vi "지진 계측기 프로젝트.vi"() -> ()   [LabVIEW 2021]
uses:
  <vilib>/Utility/sysdir.llb/System Directory Type.ctl
  <vilib>/numeric/Random Number (Range) U64.vi
panel:
  out "지진센서값출력":u64(graph)
  in  "정지":bool
  in  "알람리셋":bool
  in  "감지시작":bool
  out "알림":bool
  out "출력메시지":string
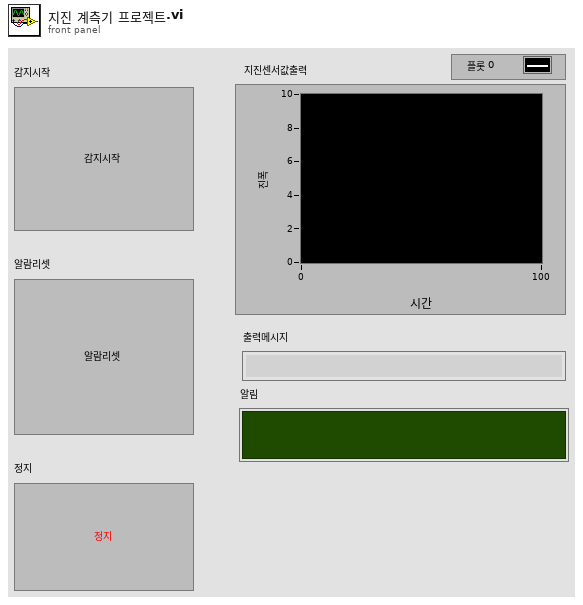
[diagram p1: front panel]
types:
  T1 = typedef "지진 계측기 상태 열거형 상수.ctl" = enum16{"초기화", "대기", "감지 시작", "알림 리셋", "정지"}
  T2 = cluster{"상태":T1, "알림":bool, "출력메시지":string, "지진센서값":dbl, "시간상수":i32}
  T3 = typedef "지진 계측기 상태 열거형 상수.ctl" = enum16{"초기화", "대기", "감지시작", "알람리셋", "정지", "파일저장"}
  T4 = enum16{"open", "replace", "create", "open or create", "replace or create", "replace or create with confirmation"}
  T5 = typedef "System Directory Type.ctl" = i32
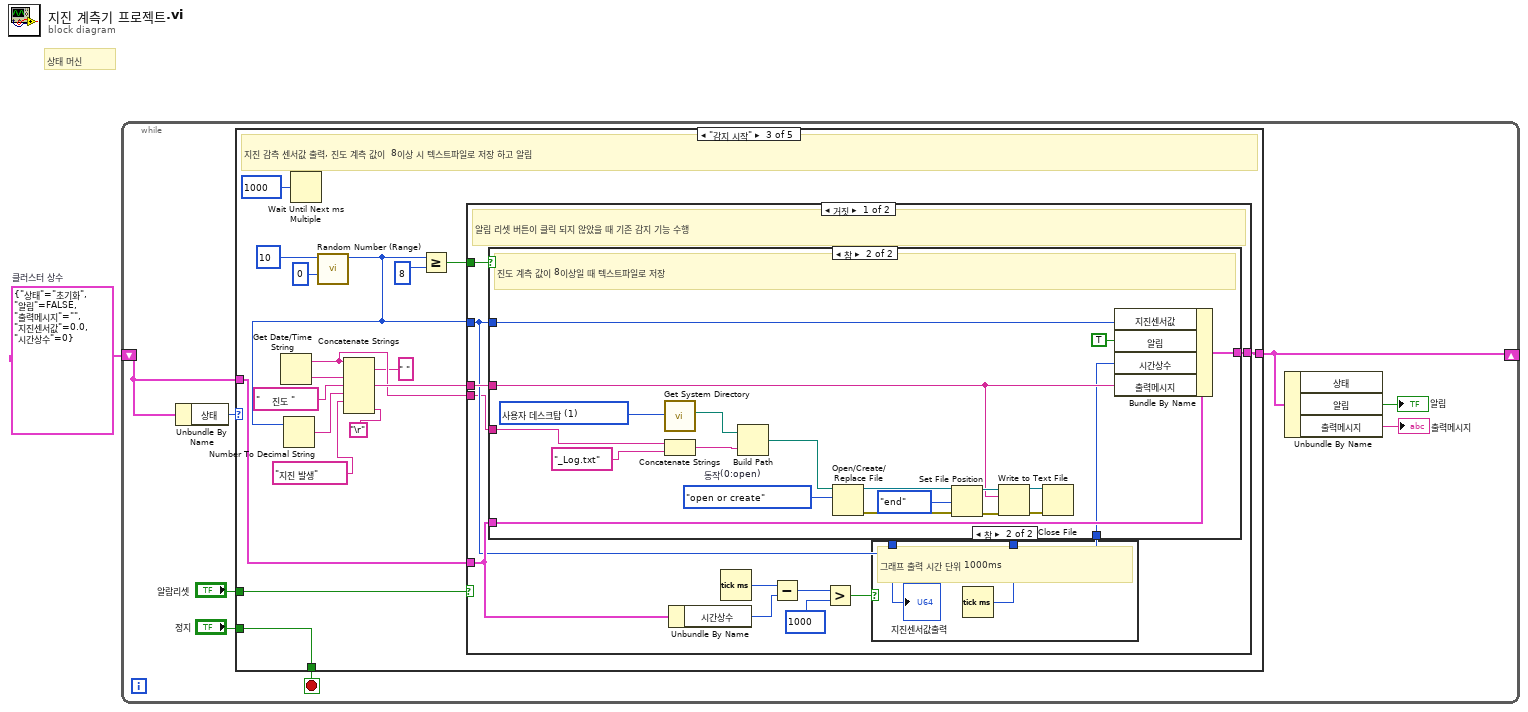
[diagram p0: block diagram]
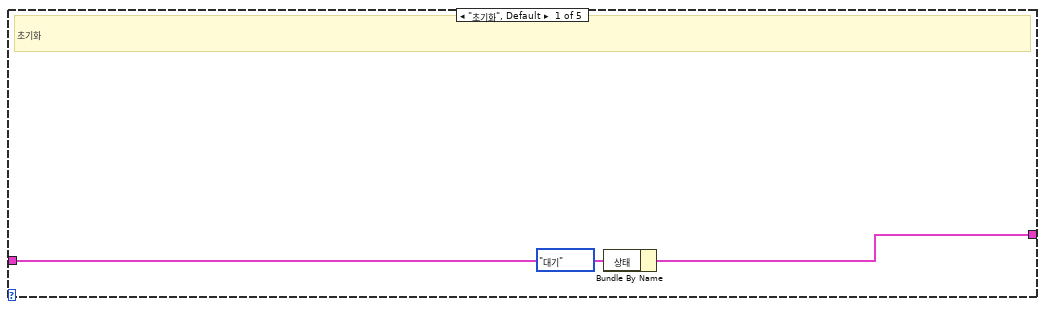
[diagram p2: hidden frame]
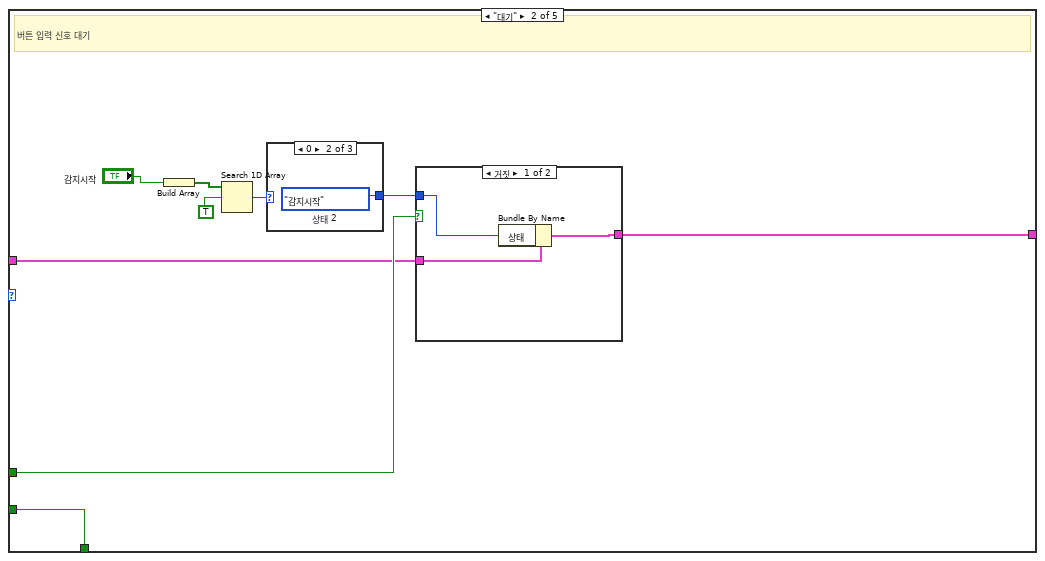
[diagram p3: hidden frame]
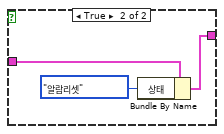
[diagram p4: hidden frame]
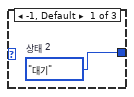
[diagram p5: hidden frame]
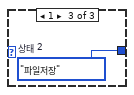
[diagram p6: hidden frame]
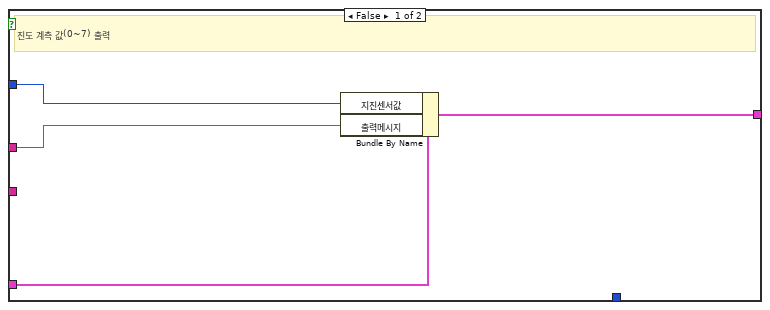
[diagram p8: hidden frame]
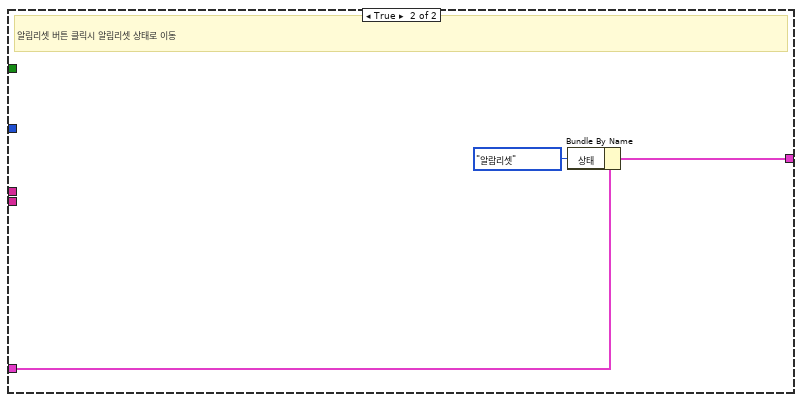
[diagram p9: hidden frame]
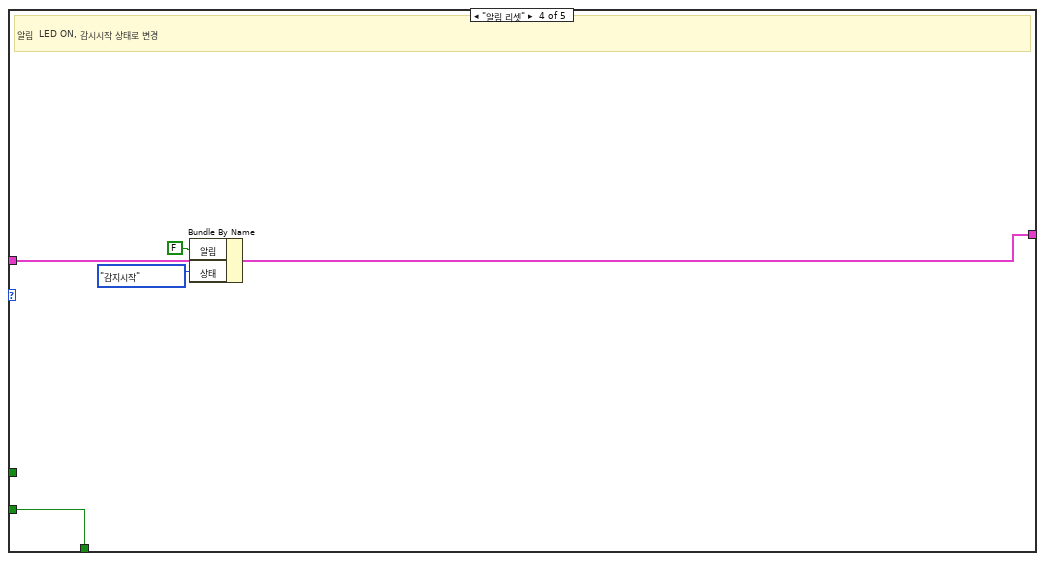
[diagram p10: hidden frame]
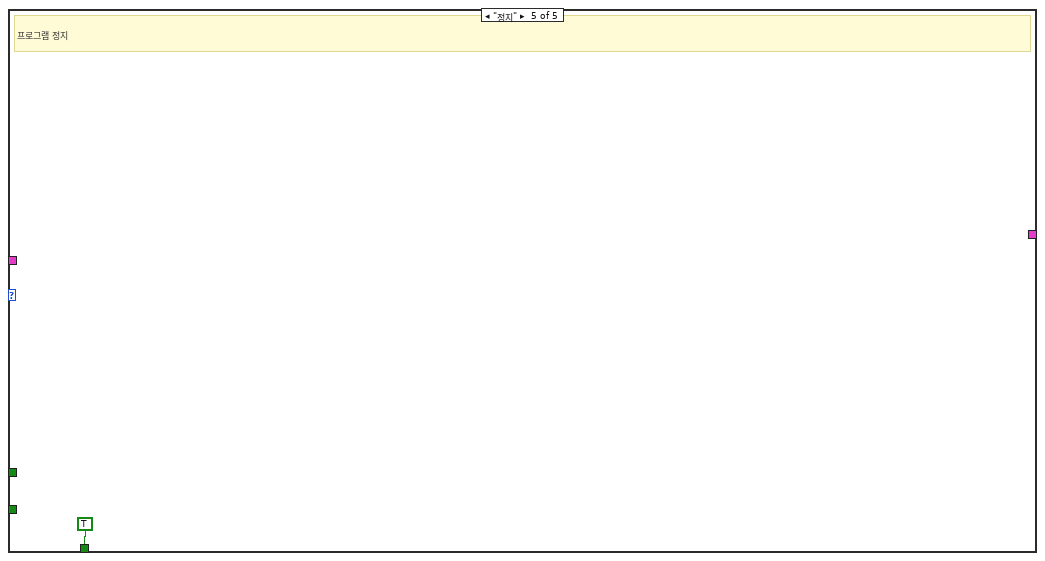
[diagram p11: hidden frame]
diagram:
  w1 = T2 {"상태"=enum."초기화", "알림"=FALSE, "출력메시지"="", "지진센서값"=0.0, "시간상수"=0}  # 클러스터 상수
  # "상태 머신"
  n1 = while {
    shift-right: [w8] -> _
    shift-left: w1 -> [w9]
    stop <- w7 stop-if-true
    n2 = Unbundle By Name(w9) -> ("상태"=w2:T1)
    n3 = case shown="\"감지 시작\"" w2 {
      tunnel: [w11 w15 w43 w91 _] -> w8
      tunnel: w9 -> [w12 w13 w42 w94 _]
      tunnel: [_ w14 w38 w90 TRUE] -> w7
      tunnel: "알람리셋" -> [_ w17 w41 _ _]
      tunnel: "정지" -> [_ w14 w38 w90 _]
      frame "초기화", Default {
        # "초기화"
        n4 = Bundle By Name(cluster=w12, "상태"=지진_계측기_상태_열거형_상수."대기") -> (w11:T2)
      }
      frame "대기" {
        # "버튼 입력 신호 대기"
        n5 = Build Array("감지시작") -> (w21:bool[])
        n6 = Search 1D Array(1D array=w21, element=TRUE ("원소")) -> (index of element=w19:i32)  [unwired: 1 in]
        n7 = case shown="0" w19 {
          tunnel: [w28 w29 w30] -> w16
          frame -1, Default {
            w28 = 지진_계측기_상태_열거형_상수."대기"  # 상태 2
          }
          frame 0 {
            w29 = 지진_계측기_상태_열거형_상수."감지시작"  # 상태 2
          }
          frame 1 {
            w30 = 지진_계측기_상태_열거형_상수."파일저장"  # 상태 2
          }
        }
        n8 = case shown="거짓" w17 {
          tunnel: w16 -> [w22 _]
          tunnel: [w23 w27] -> w15
          tunnel: w13 -> [w24 w26]
          frame False {
            n9 = Bundle By Name(cluster=w24, "상태"=w22) -> (w23:T2)
          }
          frame True {
            n10 = Bundle By Name(cluster=w26, "상태"=지진_계측기_상태_열거형_상수."알람리셋") -> (w27:T2)
          }
        }
      }
      frame "감지 시작" {
        # "지진 감측 센서값 출력, 진도 계측 값이  8이상 시 텍스트파일로 저장 하고 알림"
        n11 = Get Date/Time String() -> (date string=w37:string, time string=w32:string)  [unwired: 3 in]
        n12 = Wait Until Next ms Multiple(millisecond multiple=u32 1000 ("ms 배수")) -> ()  [unwired: 1 out]
        n13 = call-poly <vilib>:"Random Number (Range).vi"("lower bound (0)"=u64 0, "upper bound (100)"=u64 10) -> ("number"=w40:u64)  [unwired: 9 in]
        n14 = Number To Decimal String(number=w40) -> (decimal integer string=w34:string)  [unwired: 1 in]
        n15 = Concatenate Strings ("문자열 연결")(w37, " " ("문자열"), w32, "    진도 " ("문자열"), w34, "지진 발생" ("문자열"), "\r") -> (w39:string)
        n16 = Greater Or Equal?(x=w40, y=u64 8) -> (x >= y?=w44:bool)
        n17 = case shown="거짓" w41 {
          tunnel: w44 -> [w60 _]
          tunnel: [w58 w88] -> w43
          tunnel: w42 -> [w52 w89]
          tunnel: w40 -> [w50 _]
          tunnel: w39 -> [w59 _]
          tunnel: w37 -> [w49 _]
          frame False {
            # "알림 리셋 버튼이 클릭 되지 않았을 때 기존 감지 기능 수행"
            n18 = Unbundle By Name(w52) -> ("시간상수"=w56:i32)
            n19 = Tick Count (ms)() -> (millisecond timer value=w57:u32)
            n20 = Subtract(x=w57, y=w56) -> (x-y=w55:u32)
            n21 = Greater?(x=w55, y=u32 1000) -> (0:w53:bool)
            n22 = case shown="참" w53 {
              tunnel: [_ w62] -> w51
              tunnel: w50 -> [_ w61]
              frame False {
              }
              frame True {
                # "그래프 출력 시간 단위 1000ms"
                n23 = Tick Count (ms)() -> (millisecond timer value=w62:u32)
                "지진센서값출력" <- w61
              }
            }
            n24 = case shown="참" w60 {
              tunnel: w50 -> [w63 w70]
              tunnel: [w66 w73] -> w58
              tunnel: w59 -> [w65 w74]
              tunnel: w52 -> [w64 w72]
              tunnel: w51 -> [_ w71]
              tunnel: w49 -> [_ w67]
              frame False {
                # "진도 계측 값(0~7) 출력"
                n25 = Bundle By Name(cluster=w64, "지진센서값"=w63, "출력메시지"=w65) -> (w66:T2)
              }
              frame True {
                w77 = T4."open or create"  # 동작(0:open)
                w76 = T5 1 items=["사용자 홈"=0, "사용자 데스크탑"=1, "사용자 문서"=2, "사용자 어플리케이션 데이터"=3, "사용자 환경"=4, "사용자 임시"=5, "퍼블릭 문서"=6, "퍼블릭 어플리케이션 데이터"=7, "퍼블릭 환경"=8, "퍼블릭 캐시"=13, "시스템 코어 라이브러리"=9, "시스템 설치된 라이브러리"=10, "어플리케이션 파일"=11, "부팅 볼륨 루트"=12] ("system directory type")
                # "진도 계측 값이 8이상일 때 텍스트파일로 저장"
                n26 = call <vilib>:"Get System Directory.vi"("system directory type"=w76) -> ("system directory"=w75:path)  [unwired: 10 in]
                n27 = Concatenate Strings ("문자열 연결")(w67, "_Log.txt" ("문자열")) -> (w68:string)
                n28 = Build Path ("경로 만들기")(base path=w75, name or relative path=w68) -> (appended path=w85:path)
                n29 = Open/Create/Replace File ("파일 열기/생성/대체")(file path (use dialog)=w85, operation (0:open)=w77) -> (refnum out=w80:refnum<file>, error out=w79:errorcluster)  [unwired: 4 in, 1 out]
                n30 = Set File Position ("파일 위치 설정")(refnum=w80, from (0:start)=enum16{"start", "end", "current"}."end" ("위치(0:start)"), error in=w79) -> (refnum out=w82:refnum<file>, error out=w81:errorcluster)  [unwired: 1 in]
                n31 = Write to Text File ("텍스트 파일에 쓰기")(file (use dialog)=w82, text=w74, error in=w81) -> (refnum out=w84:refnum<file>, error out=w83:errorcluster)  [unwired: 1 in, 1 out]
                n32 = Close File ("파일 닫기")(refnum=w84, error in=w83) -> ()  [unwired: 2 out]
                n33 = Bundle By Name(cluster=w72, "지진센서값"=w70, "알림"=TRUE, "시간상수"=w71, "출력메시지"=w74) -> (w73:T2)
              }
            }
          }
          frame True {
            # "알림리셋 버튼 클릭시 알림리셋 상태로 이동"
            n34 = Bundle By Name(cluster=w89, "상태"=지진_계측기_상태_열거형_상수."알람리셋") -> (w88:T2)
          }
        }
      }
      frame "알림 리셋" {
        # "알림  LED ON, 감시시작 상태로 변경"
        n35 = Bundle By Name(cluster=w94, "알림"=FALSE, "상태"=지진_계측기_상태_열거형_상수."감지시작") -> (w91:T2)
      }
      frame "정지" {
        # "프로그램 정지"
      }
    }
    n36 = Unbundle By Name(w8) -> ("알림"=→"알림":bool, "출력메시지"=→"출력메시지":string)  [unwired: 1 out]
  }
